vi "Check Collision.vi"(11 "Collision in":refnum<class "Collision.lvclass">) -> (3 "Collision out":refnum<class "Collision.lvclass">, 4 "Collision?":bool, 5 "Dichotomie factor out":dbl)   [LabVIEW 2024, in "Collision.lvclass"]
doc: "MIT Licence\nCopyright (c) 2024 David Grollier"
uses:
  Collision.lvclass
  Collision.lvclass/Collision.ctl
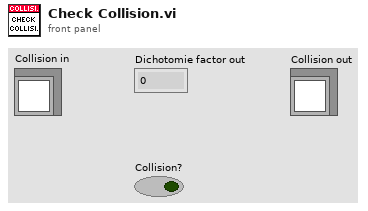
[diagram p1: front panel]
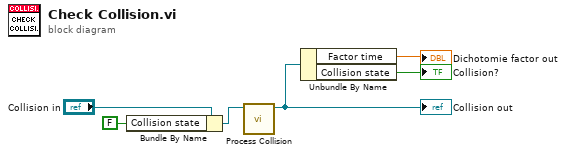
[diagram p0: block diagram]
diagram:
  n1 = Bundle By Name(cluster="Collision in", "Collision state"=FALSE) -> (w5:refnum<class "Collision.lvclass">)
  n2 = call-dynamic "Process Collision.vi"("Collision in"=w5) -> ("Collision out"=w3:refnum<class "Collision.lvclass">)  [unwired: 10 in]
  "Collision out" <- w3
  n3 = Unbundle By Name(w3) -> ("Factor time"=→"Dichotomie factor out":dbl, "Collision state"=→"Collision?":bool)
